vi "getNeighbburs.vi"(9 "col":i32, 10 "row":i32, 11 "Array":dbl[][](array[numeric])) -> (2 "neighbours":dbl[](array[numeric]), 3 "element":dbl)   [LabVIEW 2017]
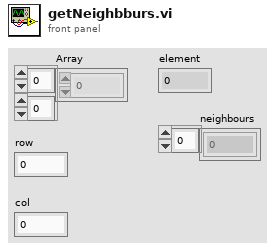
[diagram p1: front panel]
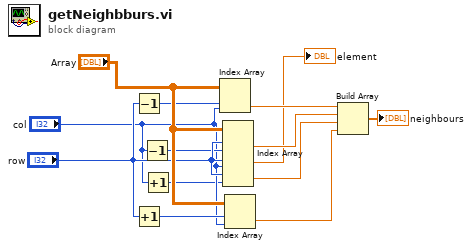
[diagram p0: block diagram]
diagram:
  n1 = Decrement(x="row") -> (x-1=w9:i32)
  n2 = Increment(x="row") -> (x+1=w7:i32)
  n3 = Decrement(x="col") -> (x-1=w8:i32)
  n4 = Increment(x="col") -> (x+1=w5:i32)
  n5 = Index Array(array="Array", index (row)=w9, index (col)="col") -> (element=w11:dbl)
  n6 = Index Array(array="Array", index (row) #1="row", index (col) #1=w8, index (row) #2="row", index (col) #2="col", index (row) #3="row", index (col) #3=w5) -> (element #1=w10:dbl, element #2=→"element":dbl, element #3=w4:dbl)
  n7 = Index Array(array="Array", index (row)=w7, index (col)="col") -> (element=w3:dbl)
  n8 = Build Array(w11, w10, w4, w3) -> (→"neighbours":dbl[])
